vi "AlazarSetCaptureClock.vi"(0 "Handle":u64, 1 "Source":u32(ring)=1 items=["Internal"=1, "Fast External"=2, "Medium External"=3, "Slow External"=4, "External AC"=5, "External DC"=6, "External 10MHz"=7], 2 "Sample Rate":u32(ring)=30 items=["1 kS/s"=1, "2 kS/s"=2, "5 kS/s"=4, "10 kS/s"=8, "20 kS/s"=10, "50 kS/s"=12, "100 kS/s"=14, "200 kS/s"=16, "500 kS/s"=18, "1 MS/s"=20, "2 MS/s"=24, "5 MS/s"=26, "10 MS/s"=28, "20 MS/s"=30, "25 MS/s"=33, "50 MS/s"=34, "100 MS/s"=36, "125 MS/s"=37, "160 MS/s"=38, "180 MS/s"=39, "250 MS/s"=43, "500 MS/s"=48, "800 MS/s"=50, "1000 MS/s"=53, "1200 MS/s"=55, "1500 MS/s"=58, "1800 MS/s"=61], 3 "Edge":u32(ring) items=["Rising", "Falling"], 4 "Decimation":u32, 5 "error in (no error)":errorcluster) -> (14 "Handle":u64, 18 "Return Code":u32, 19 "error out":errorcluster)   [LabVIEW 2018]
doc: "Configure sample clock source, edge, and decimation."
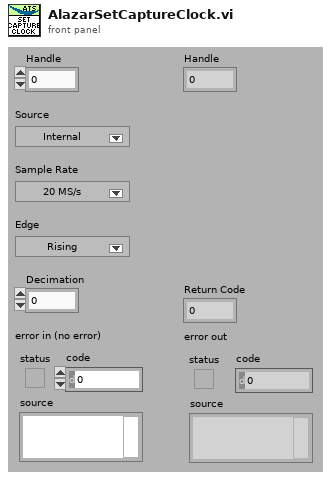
[diagram p1: front panel]
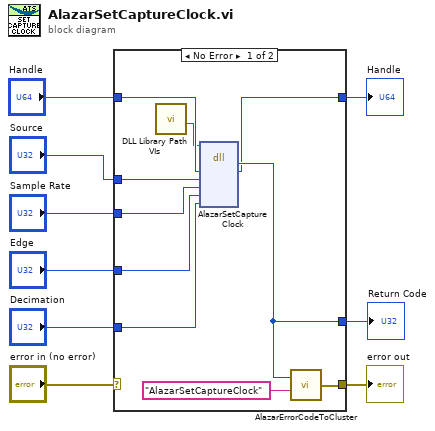
[diagram p0: block diagram]
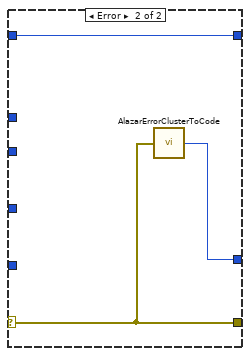
[diagram p2: hidden frame]
diagram:
  n1 = case shown="No Error" "error in (no error)" {
    selector: "error in (no error)" -> [_ w22]
    tunnel: [w16 w22] -> w8
    tunnel: [w18 w21] -> w7
    tunnel: "Handle" -> [w19 w20]
    tunnel: [w15 w20] -> w5
    tunnel: "Source" -> [w14 _]
    tunnel: "Sample Rate" -> [w13 _]
    tunnel: "Edge" -> [w12 _]
    tunnel: "Decimation" -> [w11 _]
    frame No Error {
      n2 = call "DLL Library Path VIs.vi"() -> ("Alazar"=w10:path)  [unwired: 5 in, 6 out]
      n3 = dll-call lib="C:/Project/SerialSectOCT - FFT GPU/SerialSectOCT/Labview Software/DLL/ATSApi.dll" fn="AlazarSetCaptureClock"(path in=w10, "handle"=w19, "source"=w14, "sampleRate"=w13, "edge"=w12, "decimation"=w11) -> ("return type"=w18:u32, "handle"=w15:u64)  [unwired: 6 in, 2 out]
      n4 = call "AlazarErrorCodeToCluster.vi"("Message"="AlazarSetCaptureClock", "Error Code"=w18) -> ("error out"=w16:errorcluster)
    }
    frame Error {
      n5 = call "AlazarErrorClusterToCode.vi"("error in (no error)"=w22) -> ("Error Code"=w21:u32)
    }
  }
  "Handle" <- w5
  "error out" <- w8
  "Return Code" <- w7
